vi "Test Request Read Data.vi"() -> ()   [LabVIEW 2014]
uses:
  ALPHA5 RS485/typedefs/Port Selection Info.ctl
  ALPHA5 RS485/ALPHA5 RS485.lvlib
panel:
  out "Data":u32[](array[numeric])
  out "Received Read Data":u8[](array[numeric]) format="%.0x"
  out "CRC Check?":bool
  out "Time Out?":bool
  out "error out":errorcluster
  in  "Wait Time(ms)":u32=50
  in  "Specified Num in":u8=1
  in  "Address":u16=4102 format="%.0x"
  in  "error in (no error)":errorcluster caption="error in（no error）"
  in  "Port Selection Info In":T1={"Port Name"="", "Amplifier Num"=1, "Baud Rate"=38400, "Char Formation"=enum."0"} {"Baud Rate" items=["38400"=38400, "19200"=19200, "9600"=9600, "115200"=0]; "Amplifier Num" max=31}
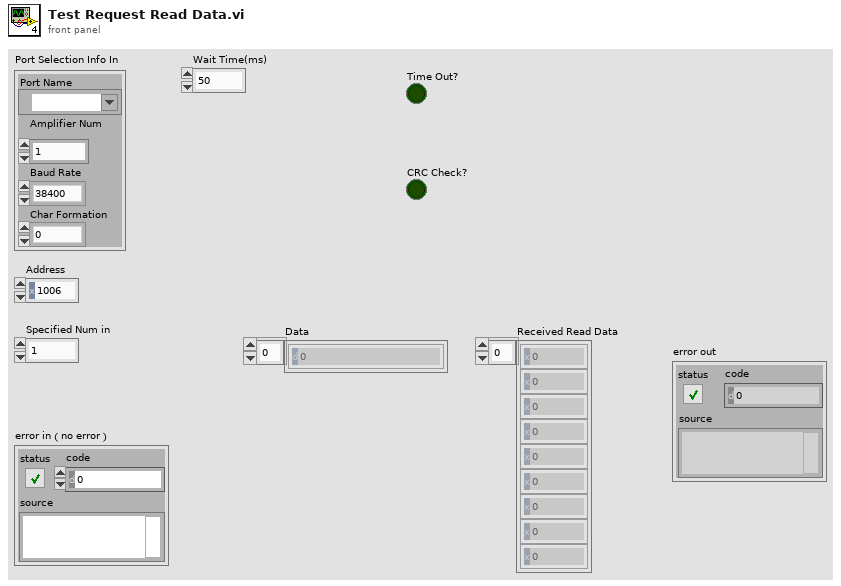
[diagram p1: front panel]
types:
  T1 = typedef "ALPHA5 RS485.lvlib/Port Selection Info.ctl" = cluster{"Port Name":refnum<visa-resource-name>, "Amplifier Num":u8, "Baud Rate":u32, "Char Formation":enum16{"0", "1", "2", "3", "4", "5"}}
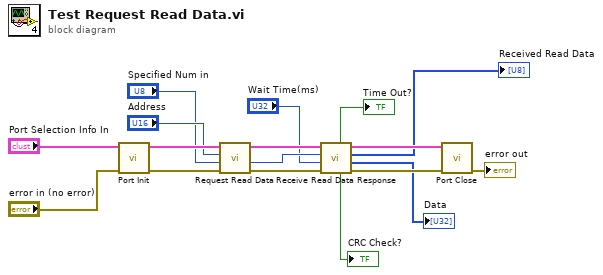
[diagram p0: block diagram]
diagram:
  n1 = call "Port Init.vi"("error in (no error)"="error in (no error)", "Port Selection Info In"="Port Selection Info In") -> ("error out"=w13:errorcluster, "Port Selection Info Out"=w16:T1)  [unwired: 8 in]
  n2 = call "Request Read Data.vi"("error in (no error)"=w13, "Specified Num in"="Specified Num in", "Address"="Address", "Port Selection Info"=w16) -> ("error out"=w8:errorcluster, "Specified Num out"=w10:u8, "Port Selection Info Out"=w11:T1)  [unwired: 5 in]
  n3 = call "Receive Read Data Response.vi"("error in (no error)"=w8, "Wait Time(ms)"="Wait Time(ms)", "Specified Num in"=w10, "Port Selection Info"=w11) -> ("error out"=w6:errorcluster, "Data"=→"Data":u32[], "Received Read Data"=→"Received Read Data":u8[], "Port Selection Info Out"=w7:T1, "CRC Check?"=→"CRC Check?":bool, "Time Out?"=→"Time Out?":bool)  [unwired: 2 in]
  n4 = call "Port Close.vi"("error in (no error)"=w6, "Port Selection Info In"=w7) -> ("error out"=→"error out":errorcluster)  [unwired: 9 in]
